vi "SequenceIndexCheck.vi"(8 "error in (no error)":errorcluster, 9 "OriginalName":string, 10 "SequenceIndex":refnum<class "SequenceIndex.lvclass">, 11 "VariableManagerRef in":refnum<vi>) -> (0 "error out":errorcluster, 1 "RejectMessage":string, 2 "Pass":bool=TRUE, 3 "VariableManagerRef out":refnum<vi>)   [LabVIEW 2012, in "VariableManagerAPI.lvlib"]
doc: "Check the given sequence index definition before adding to database.\n\nReturn true if the given sequence index passes all tests.\nReturn false if the given sequence index fails some tests.\nRejectMessage can be used to identify the failed tests. \n\nThe following will make a sequence index definition fails the test:\n1. The difinition has an empty name\n2. Steps is less than 1\n3. The name is already used by another sequence index. Providing OriginalName will bypass the check against the given OriginalName\n4. The name is already used by another variable.\n5. The name begins with number.\n6. The name is t or f (reserved variable name)"
uses:
  VariableManagerAPI.lvlib
  VariableManager/VariableManager.lvclass
  SequenceIndex/SequenceIndex.lvclass
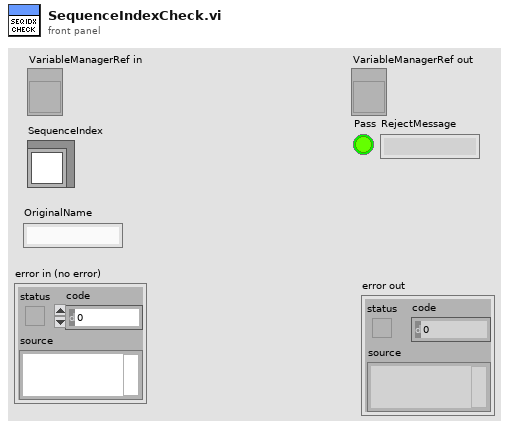
[diagram p1: front panel]
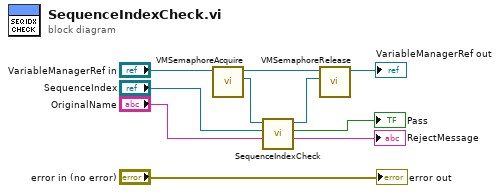
[diagram p0: block diagram]
diagram:
  n1 = call "VMSemaphoreAcquire.vi"("VariableManagerRef in"="VariableManagerRef in") -> ("VariableManager"=w6:refnum<class "VariableManager.lvclass">, "VariableManagerRef out"=w9:refnum<vi>)  [unwired: 7 in, 2 out]
  n2 = call-dynamic "SequenceIndexCheck.vi"("OriginalName"="OriginalName", "SequenceIndex"="SequenceIndex", "VariableManager in"=w6) -> ("RejectMessage"=→"RejectMessage":string, "Pass"=→"Pass":bool, "VariableManager out"=w5:refnum<class "VariableManager.lvclass">)  [unwired: 5 in, 1 out]
  n3 = call "VMSemaphoreRelease.vi"("VariableManager"=w5, "VariableManagerRef in"=w9) -> ("VariableManagerRef out"=→"VariableManagerRef out":refnum<vi>)  [unwired: 8 in, 1 out]
  "error out" <- "error in (no error)"
